vi "Get ChnlHits Semaphore.vi"(8 "error in (no error)":errorcluster) -> (0 "error out":errorcluster, 2 "timed out":bool, 3 "Refnum out":T1)   [LabVIEW 2016]
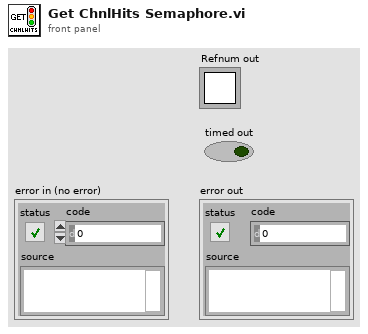
[diagram p1: front panel]
types:
  T1 = typedef "Semaphore RefNum" = refnum<k1>
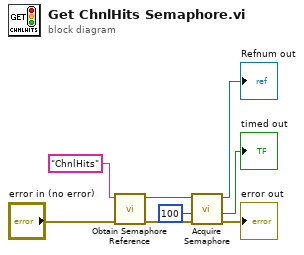
[diagram p0: block diagram]
diagram:
  n1 = call <vilib>:"Obtain Semaphore Reference.vi"("error in (no error)"="error in (no error)", "name (unnamed)"="ChnlHits") -> ("error out"=w3:errorcluster, "semaphore"=w2:T1)  [unwired: 3 in, 1 out]
  n2 = call <vilib>:"Acquire Semaphore.vi"("error in (no error)"=w3, "ms timeout (-1)"=100, "semaphore"=w2) -> ("error out"=→"error out":errorcluster, "timed out"=→"timed out":bool, "semaphore out"=→"Refnum out":T1)  [unwired: 2 in]
